vi "Obtain System Ref.vi"(8 "error in (no error)":errorcluster) -> (0 "error out":errorcluster, 3 "JKI SMO System":refnum<data-value>)   [LabVIEW 2021, in "smo.lvlib" / "Registry-SMO.lvclass"]
uses:
  Registry-SMO.lvclass
  SMO_Info--Cluster.ctl
  Registry-SMO.lvclass/Registry-SMO.ctl
  Support/Attribute.Identity/Attribute.Identity.lvclass
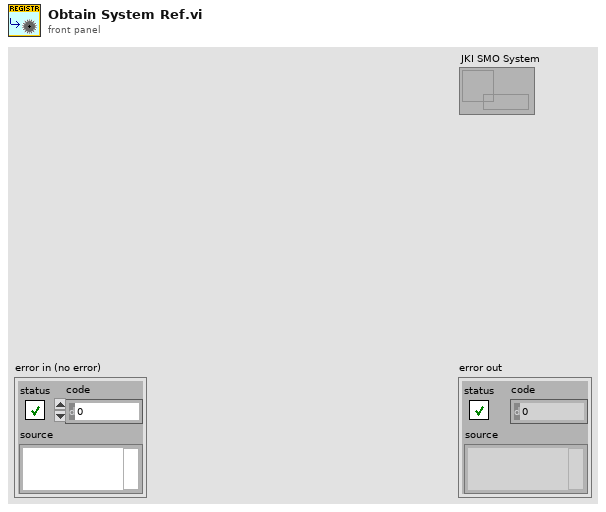
[diagram p1: front panel]
types:
  T1 = typedef "smo.lvlib/Registry-SMO.lvclass/SMO_Info--Cluster.ctl" = cluster{"Name":string, "Shared Resource":bool}
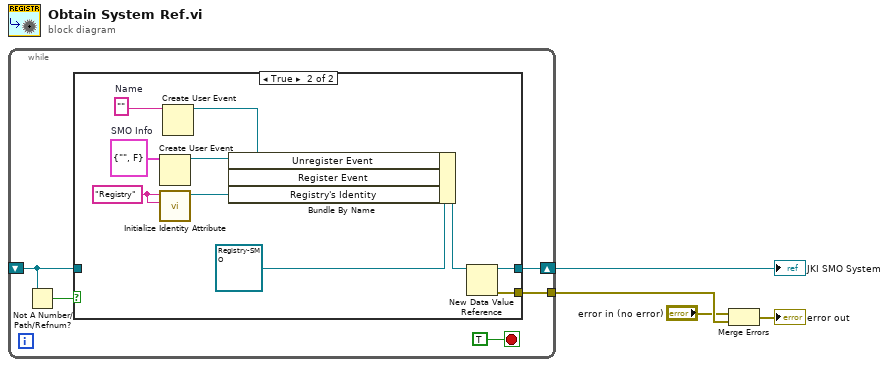
[diagram p0: block diagram]
diagram:
  n1 = while {
    shift-right: [w9] -> w4
    shift-left: _ -> [w6]
    tunnel: [w5] -> w3
    stop <- TRUE stop-if-true
    n2 = Not A Number/Path/Refnum?(number/path/refnum=w6) -> (NaN/Path/Refnum?=w7:bool)
    n3 = case shown="True" w7 {
      tunnel: [w10 w20] -> w9
      tunnel: w6 -> [w10 _]
      tunnel: [_ w19] -> w5
      frame False {
      }
      frame True {
        w13 = ""  # Name
        w18 = T1 {"Name"="", "Shared Resource"=FALSE}  # SMO Info
        w11 = "Registry" ("Name")
        n4 = Create User Event(user event datatype=w18) -> (user event=w14:refnum<user-event>)  [unwired: 1 in, 1 out]
        n5 = call "Initialize Identity Attribute.vi"("Unique Name"=w11, "Given Name"=w11) -> ("Attribute.Identity"=w17:refnum<class "Attribute.Identity.lvclass">)  [unwired: 8 in, 1 out]
        n6 = Create User Event(user event datatype=w13) -> (user event=w12:refnum<user-event>)  [unwired: 1 in, 1 out]
        n7 = Bundle By Name(cluster=refnum<class "Registry-SMO.lvclass"> refnum ("JKI SMO System"), "Unregister Event"=w12, "Register Event"=w14, "Registry's Identity"=w17) -> (w15:refnum<class "Registry-SMO.lvclass">)
        n8 = New Data Value Reference(data value=w15) -> (data value reference=w20:refnum<data-value>, error out=w19:errorcluster)  [unwired: 1 in]
      }
    }
  }
  "JKI SMO System" <- w4
  n9 = Merge Errors("error in (no error)", w3) -> (→"error out":errorcluster)
